vi "PH_Beckhoff_PP_PU.set i Attr and start DIM Services for  HV Meas.vi"(3 "error in":errorcluster, 4 "Values":T3, 5 "PU Type":T2=enum."PA 19mm") -> (0 "error out":errorcluster, 1 "HV Meas":T1(array[cluster]))   [LabVIEW 2014, in "PH_Beckhoff_PP_PU.lvlib"]
uses:
  PH_Beckhoff_PP_PU.lvlib
  PH_Beckhoff/PH_Beckhoff.Values.ctl
  PH_Beckhoff/PH_Beckhoff.Sonderklemmen Inputs.ctl
  PH_Beckhoff/PH_Beckhoff.Analog Inputs.ctl
  PH_Beckhoff/PH_Beckhoff.Scaling Type.ctl
  PH_Beckhoff/PH_Beckhoff.Analog Outputs.ctl
  PH_Beckhoff/PH_Beckhoff.Digital Inputs.ctl
  PH_Beckhoff/PH_Beckhoff.Digital Outputs.ctl
  PH_Beckhoff_PP_PU.PU Rack Type.ctl
  PH_Beckhoff_PP_PU.HV Meas Tags.ctl
  lib.lib/DimLVEvent/LVDimInterface/LVDimInterface.lvlib
  PH_Beckhoff/PH_Beckhoff.lvlib
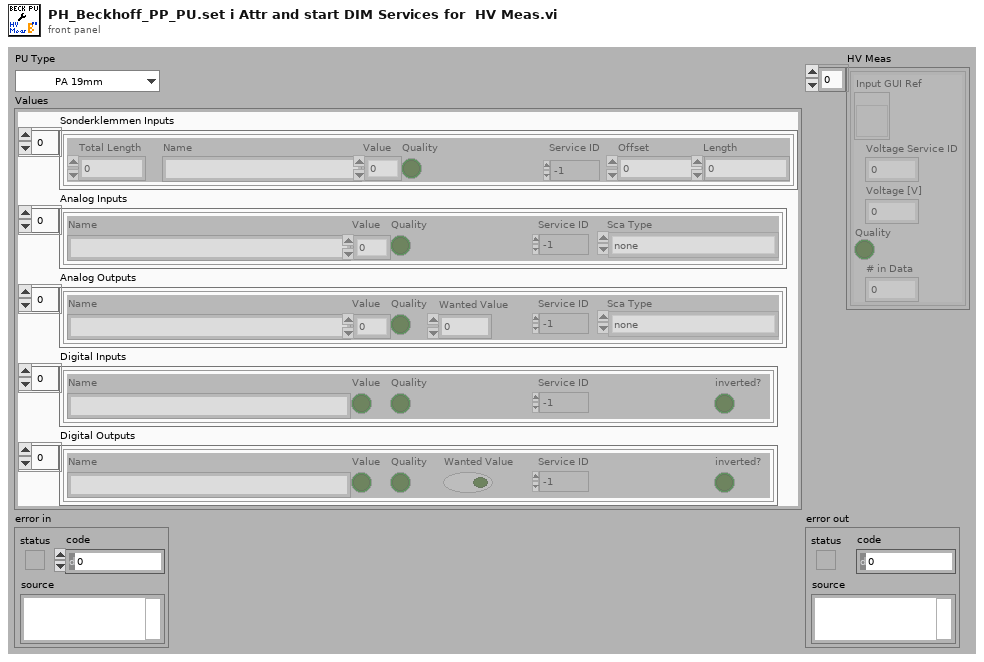
[diagram p1: front panel]
types:
  T1 = cluster{"Input GUI Ref":refnum<vi>, "Voltage Service ID":i32, "Voltage [V]":dbl, "Quality":bool, "# in Data":i32}[]
  T2 = typedef "PH_Beckhoff_PP_PU.lvlib/PH_Beckhoff_PP_PU.PU Rack Type.ctl" = enum16{"no Info", "PA 19mm", "PA 45mm", "MA PU 1 and 2", "MA PU 3 and 4", "MA PU 5 and 6", "MA FR and PILC"}
  T3 = typedef "PH_Beckhoff.lvlib/PH_Beckhoff.Values.ctl" = cluster{"Sonderklemmen Inputs":T4, "Analog Inputs":T5, "Analog Outputs":T7, "Digital Inputs":T8, "Digital Outputs":T9}
  T4 = typedef "PH_Beckhoff.lvlib/PH_Beckhoff.Sonderklemmen Inputs.ctl" = cluster{"Total Length":u32, "Name":string, "Value":u64, "Quality":bool, "Service ID":i32, "Offset":u32, "Length":u32}[]
  T5 = typedef "PH_Beckhoff.lvlib/PH_Beckhoff.Analog Inputs.ctl" = cluster{"Name":string, "Value":u32, "Quality":bool, "Service ID":i32, "Sca Type":T6}[]
  T6 = typedef "PH_Beckhoff.lvlib/PH_Beckhoff.Scaling Type.ctl" = enum16{"none", "0 ... 15 Bit -> 0 ... 5", "0 ... 15 Bit -> 0 ... 10", "0 ... 15 Bit -> 0 ... 25", "0 ... 15 Bit -> 4 ... 20", "0 ... 15 Bit -> 0 ... 1", "0 ... 15 Bit -> 0 ... 20000", "0 ... 15 Bit -> 0 ... 24000"}
  T7 = typedef "PH_Beckhoff.lvlib/PH_Beckhoff.Analog Outputs.ctl" = cluster{"Name":string, "Value":u32, "Quality":bool, "Wanted Value":u32, "Service ID":i32, "Sca Type":T6}[]
  T8 = typedef "PH_Beckhoff.lvlib/PH_Beckhoff.Digital Inputs.ctl" = cluster{"Name":string, "Value":bool, "Quality":bool, "Service ID":i32, "inverted?":bool}[]
  T9 = typedef "PH_Beckhoff.lvlib/PH_Beckhoff.Digital Outputs.ctl" = cluster{"Name":string, "Value":bool, "Quality":bool, "Wanted Value":bool, "Service ID":i32, "inverted?":bool}[]
  T10 = typedef "PH_Beckhoff_PP_PU.lvlib/PH_Beckhoff_PP_PU.HV Meas Tags.ctl" = enum16{"voltage-raw", "voltage"}
  T11 = typedef "PH_PP_Common.lvlib/PH_PP_Common.PUs.ctl" = enum16{"no Info", "PA-19mm-1", "PA-19mm-2", "PA-45mm-PILC", "PA-45mm-MAIN", "MA-PU-1", "MA-PU-2", "MA-PU-3", "MA-PU-4", "MA-PU-5", "MA-PU-6", "MA-FR", "MA-PILC", "PA-45mm-DP"}
  T12 = cluster{"Input GUI Ref":refnum<vi>, "Voltage Service ID":i32, "Voltage [V]":dbl, "Quality":bool, "# in Data":i32}
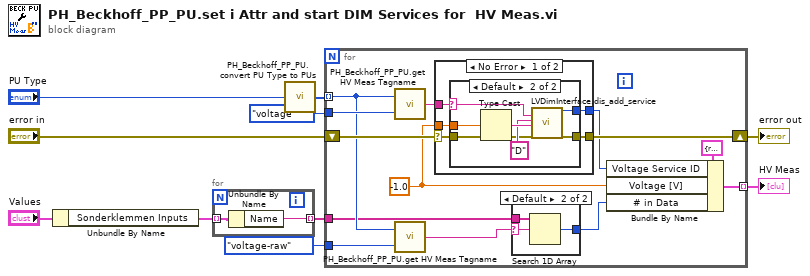
[diagram p0: block diagram]
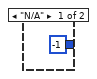
[diagram p2: hidden frame]
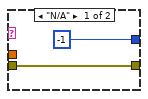
[diagram p3: hidden frame]
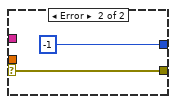
[diagram p4: hidden frame]
diagram:
  n1 = Unbundle By Name("Values") -> ("Sonderklemmen Inputs"=w5:T4)
  n2 = for {
    tunnel: w5 -> [w12] mode=indexing
    tunnel: [w11] -> w4 mode=indexing
    n3 = Unbundle By Name(w12) -> ("Name"=w11:string)
  }
  n4 = call "PH_Beckhoff_PP_PU.convert PU Type to PUs.vi"("PU Type"="PU Type") -> ("PUs"=w7:T11[])
  n5 = for {
    shift-right: [w23] -> w10
    shift-left: "error in" -> [w24]
    tunnel: [w25] -> w2 mode=indexing
    tunnel: w7 -> [w18] mode=indexing
    tunnel: PH_Beckhoff_PP_PU.HV_Meas_Tags."voltage" ("HV Meas Tag") -> [w19]
    tunnel: w4 -> [w15]
    tunnel: PH_Beckhoff_PP_PU.HV_Meas_Tags."voltage-raw" ("HV Meas Tag") -> [w17]
    w21 = -1.0 ("Double Value")
    n6 = call "PH_Beckhoff_PP_PU.get HV Meas Tagname.vi"("HV Meas Tag"=w19, "PU"=w18) -> ("HV Meas Tagname"=w22:string)
    n7 = call "PH_Beckhoff_PP_PU.get HV Meas Tagname.vi"("HV Meas Tag"=w17, "PU"=w18) -> ("HV Meas Tagname"=w16:string)
    n8 = case shown="No Error" w24 {
      selector: w24 -> [w32 w45]
      tunnel: [w34 -1 ("my_serviceID")] -> w20
      tunnel: [w33 w45] -> w23
      tunnel: w21 -> [w31 _]
      tunnel: w22 -> [w30 _]
      frame No Error {
        n9 = case shown="Default" w30 {
          selector: w30 -> [_ w37]
          tunnel: [-1 ("my_serviceID") w39] -> w34
          tunnel: [w36 w40] -> w33
          tunnel: w32 -> [w36 w41]
          tunnel: w31 -> [_ w38]
          frame "N/A" {
          }
          frame Default {
            n10 = Type Cast(x=w38) -> (*(type *) &x=w43:string)  [unwired: 1 in]
            n11 = call "LVDimInterface.dis_add_service.vi"("serviceName"=w37, "typeDescriptor"="D", "data"=w43, "error in (no error)"=w41) -> ("my_serviceID"=w39:i32, "error out"=w40:errorcluster)  [unwired: 14 in]
          }
        }
      }
      frame Error {
      }
    }
    n12 = case shown="Default" w16 {
      selector: w16 -> [_ w27]
      tunnel: [-1 ("my_serviceID") w29] -> w14
      tunnel: w15 -> [_ w28]
      frame "N/A" {
      }
      frame Default {
        n13 = Search 1D Array(1D array=w28, element=w27) -> (index of element=w29:i32)  [unwired: 1 in]
      }
    }
    n14 = Bundle By Name(cluster=T12 {"Input GUI Ref"=refnum, "Voltage Service ID"=0, "Voltage [V]"=0.0, "Quality"=FALSE, "# in Data"=0} ("HV Meas Data"), "Voltage Service ID"=w20, "Voltage [V]"=w21, "# in Data"=w14) -> (w25:T12)
  }
  "error out" <- w10
  "HV Meas" <- w2
